vi "narrowband_response.vi"() -> ()   [LabVIEW 2012]
uses:
  Trace controls.ctl
  probe_point.ctl
  <vilib>/Analysis/4window.llb/windowTd.ctl
  stimulus.ctl
  injection_point.ctl
  pose_selector.ctl
  pose_source.ctl
  pose_relative_to.ctl
  scan_info.ctl
  <vilib>/Platform/TimedLoop/XDataNode/timing_clust.ctl
  <vilib>/Platform/TimedLoop/XDataNode/nitl_modes.ctl
  <vilib>/Platform/TimedLoop/XDataNode/wakeup.ctl
  initialization/micron_globals.vi
  <vilib>/Analysis/0measdsp.llb/Scaled Time Domain Window (DBL).vi
  <vilib>/Analysis/2dsp.llb/Real FFT.vi
  <vilib>/Analysis/2dsp.llb/Inverse Real FFT.vi
  <vilib>/Platform/TimedLoop/XDataNode/XDataNode.xnode
  <vilib>/Platform/TimedLoop/XDataNode/XDNodeRunTimeDep.lvlib
  <vilib>/Analysis/NI_AALPro.lvlib
  <vilib>/Analysis/4window.llb/Window Properties by Name.vi
  <vilib>/Analysis/4window.llb/Blackman-Harris Window (DBL).vi
panel:
  in  "Pose selectors":T1[](array[typedef])
  in  "Unwrap phase":bool=TRUE
  in  "Responses":cluster{"Individual":bool, "Vector sum":bool}={"Individual"=FALSE, "Vector sum"=TRUE}
  out "Stimulus":T4={"Type"=enum."Off", "Phase"=0.0, "Amplitude"=[0.0, 0.0, 0.0, 0.0, 0.0, 0.0], "Injection point"=enum."Total pose", "Closed loop"=FALSE, "Offset"=[0.0, 0.0, 0.0, 0.0, 0.0, 0.0], "Tip -> world"=TRUE, "Frequency"=0.0, "Length"=0.0} {"Length" min=0.0 max=100.0 step=100.0 format="%#_4p"; "Frequency" min=0.0 step=100.0 format="%#_4g"; "Offset" format="%#_3p"; "Amplitude" format="%#_3p"; "Phase" min=-180.0 max=360.0 step=100.0 format="%#.2f"}
  in  "Clear plot":bool
  out "Phase plot":T6(graph)
  out "Amplitude plot":cluster{"X out":dbl[], dbl[]}[](graph)
  out "dB re. 1 um peak":dbl caption="dB re. 1mm peak" format="%#_3f"
  out "Amplitude dB":dbl caption="dB" format="%#_3f"
  out "RMS":dbl format="%#_3p"
  out "Phase":dbl format="%#.2f"
  out "THD":dbl format="%#_4p"
  in  "N harmonics":i32=10 min=1 max=100
  out "Amplitudes":cluster{dbl, i32, dbl}[](array[cluster]) {"?" format="%#.1f"; "?" format="%#_4g"}
  in  "stop":bool
  out "Vector sum":sgl format="%#_3p"
  out "RMS":sgl[](array[numeric]) format="%#_3p"
  out "Spectrum":waveform(sgl)[](graph)
  in  "Reference":bool
  in  "Window":T7 items=["Rectangle"=0, "Hanning"=1, "Hamming"=2, "Blackman-Harris"=3, "Exact Blackman"=4, "Blackman"=5, "Flat Top"=6, "4 Term B-Harris "=7, "7 Term B-Harris"=8, "Low Sidelobe"=9, "Blackman Nuttall"=11, "Triangle"=30, "Bartlett-Hanning"=31, "Bohman"=32, "Parzen"=33, "Welch"=34, "Kaiser"=60, "Dolph-Chebyshev"=61, "Gaussian"=62]
  in  "High cutoff":sgl=100.0
  out "Time domain result":waveform(sgl)[](graph)
  in  "Components":T8={"Fundamental"=TRUE, "Harmonics"=TRUE, "Noise"=FALSE}
  out "Status":string
  in  "Trace controls":T9[](array[typedef])=[{"+ stim"=FALSE, "Relative"=FALSE, "Scale"=enum."1X", "Probe point"=enum."Position (tip)", "XYZ selector"={"Boolean"=FALSE, "Boolean 2"=FALSE, "Boolean 3"=FALSE}, "To tip"=FALSE}, {"+ stim"=FALSE, "Relative"=FALSE, "Scale"=enum."1X", "Probe point"=enum."Position (tip)", "XYZ selector"={"Boolean"=FALSE, "Boolean 2"=FALSE, "Boolean 3"=FALSE}, "To tip"=FALSE}, {"+ stim"=FALSE, "Relative"=FALSE, "Scale"=enum."1X", "Probe point"=enum."Position (tip)", "XYZ selector"={"Boolean"=FALSE, "Boolean 2"=FALSE, "Boolean 3"=FALSE}, "To tip"=FALSE}, {"+ stim"=FALSE, "Relative"=FALSE, "Scale"=enum."1X", "Probe point"=enum."Position (tip)", "XYZ selector"={"Boolean"=FALSE, "Boolean 2"=FALSE, "Boolean 3"=FALSE}, "To tip"=FALSE}]
  # "Fundamental"
  # "dB"
  # "Harmonic"
  # "Hz"
  # "Harmonics"
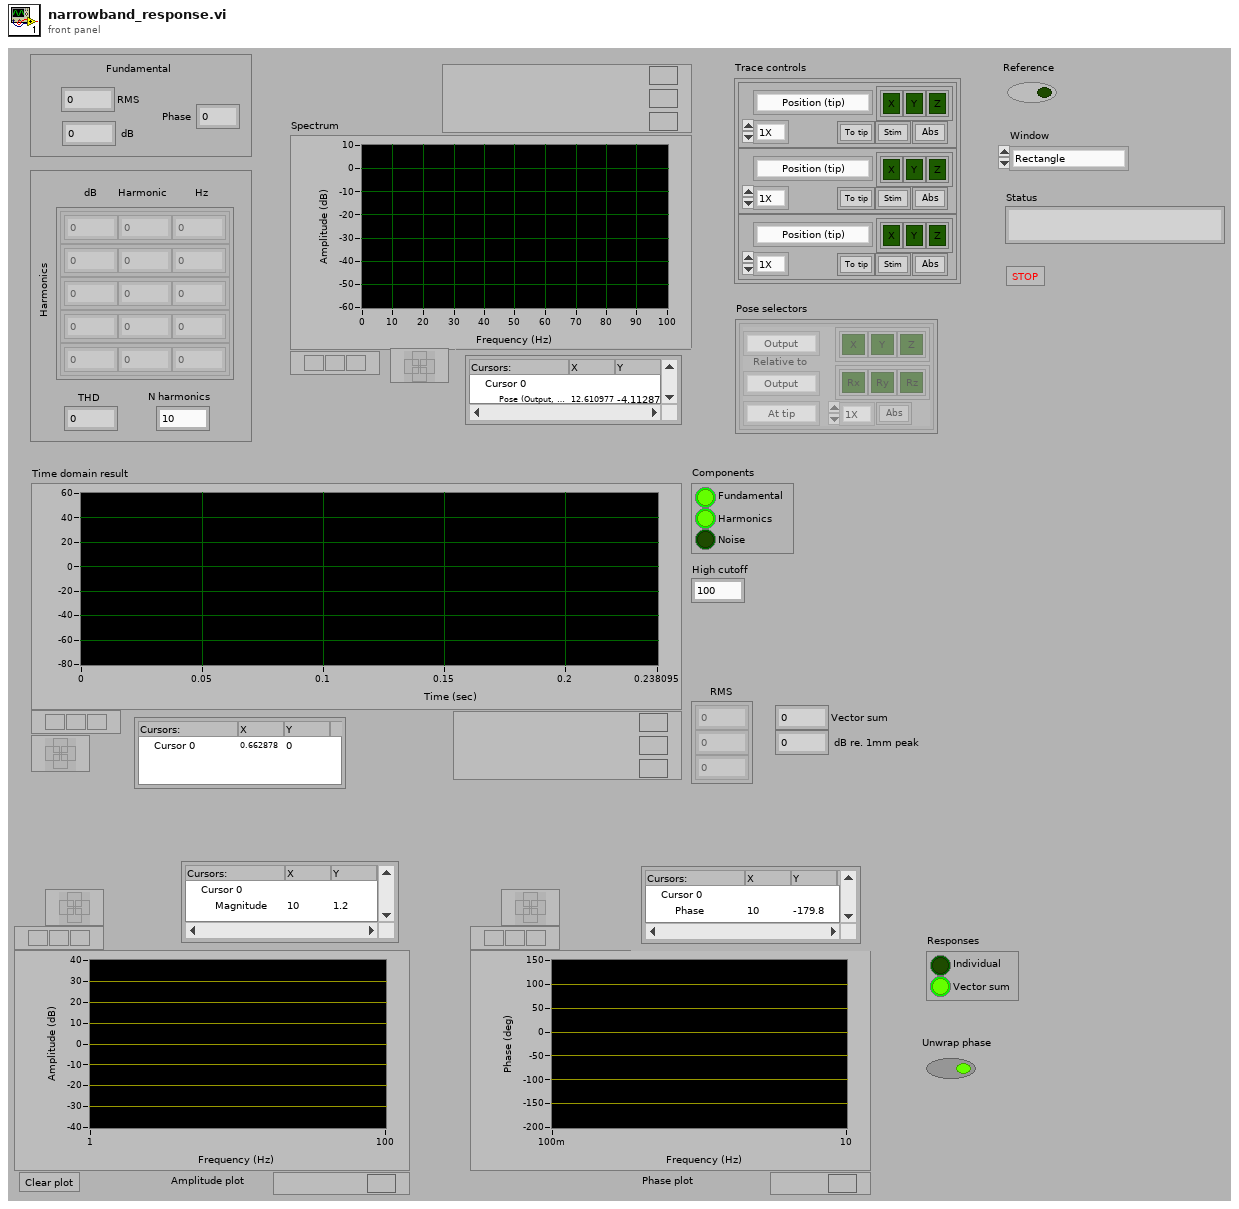
[diagram p1: front panel]
types:
  T1 = typedef "pose_selector.ctl" = cluster{"Scale":enum16{"1X", "10X", "100X", "1KX", "10KX"}, "Source":T2, "XYZ selector":cluster{"Boolean":bool, "Boolean 2":bool, "Boolean 3":bool}, "RPY selector":cluster{"Boolean":bool, "Boolean 2":bool, "Boolean 3":bool}, "Relative to":T3, "Relative":bool, "Translate":enum16{"At tip", "At RCM", "At KC", "At origin"}}
  T2 = typedef "pose_source.ctl" = enum16{"Output", "Handle", "Handle KF", "Goal", "Absolute"}
  T3 = typedef "pose_relative_to.ctl" = enum16{"Output", "Handle", "Handle KF", "Goal", "Absolute", "Trace start"}
  T4 = typedef "stimulus.ctl" = cluster{"Type":enum16{"Off", "Step", "Sine", "Triangle", "Arbitrary"}, "Phase":dbl, "Amplitude":sgl[], "Injection point":T5, "Closed loop":bool, "Offset":sgl[], "Tip -> world":bool, "Frequency":dbl, "Length":dbl}
  T5 = typedef "injection_point.ctl" = enum16{"Total pose", "V limiter", "Goal ", "Link position", "KF link position", "Inverse kin", "Link goal", "Link error", "Controller", "Output", "Drive", "Light"}
  T6 = cluster{"X out":dbl[], "Unwrapped Phase":dbl[]}[]
  T7 = typedef "NI_AALPro.lvlib/windowTd.ctl" = u32
  T8 = cluster{"Fundamental":bool, "Harmonics":bool, "Noise":bool}
  T9 = typedef "Trace controls.ctl" = cluster{"+ stim":bool, "Relative":bool, "Scale":enum16{"1X", "10X", "100X", "1KX", "10KX"}, "Probe point":T10, "XYZ selector":cluster{"Boolean":bool, "Boolean 2":bool, "Boolean 3":bool}, "To tip":bool}
  T10 = typedef "probe_point.ctl" = enum16{"Position (tip)", "Position (RCM)", "Null pos (tip)", "Null pos (RCM)", "V limiter (tip)", "V Limiter (RCM)", "Goal (tip)", "Goal (RCM)", "Link pos 0", "Link pos 1", "KF link pos 0", "KF link pos 1", "Link rate 0", "Link rate 1", "Link residue 0", "Link residue 1", "Link goal 0", "Link goal 1", "Rate limit 0", "Rate limit 1", "Link error 0", "Link error 1", "Controller 0", "Controller 1", "Output 0", "Output 1", "Drive 0", "Drive 1", "Stimulus 0", "Stimulus 1", "Trace data 0", "Trace data 1", "Analog data 0", "Analog data 1", "Status flags", "Light 0", "Light 1", "Light 2", "Light 3", "Light 4", "Light 5", "Goal origin", "Goal rotation 0", "Goal rotation 1", "Goal rotation 2", "Output origin", "Output rotation 0", "Output rotation 1", "Output rotation 2", "Handle origin", "Handle rotation 0", "Handle rotation 1", "Handle rotation 2", "Handle position", "Handle velocity", "Handle acceleration", "Handle angles", "Handle angle rates", "Handle pos residue", "Handle angle residue", "Trace length"}
  T11 = typedef "scan_info.ctl" = cluster{"Type":enum16{"Frequency", "Offset", "Motion"}, "Start":sgl, "End":sgl, "Npoints":i32}
  T12 = typedef "Micron params.ctl" = cluster{"Stimulus":T4, "Goal Filter A":T13, "Mode controls":T14, "Manipulator type":enum16{"Current piezo", "Voltage piezo"}, "Manipulator calibration":T15, "Network":T17, "Goal Filter B":T13, "Cancellation":T18, "Transition time":sgl, "Estimation":T20}
  T13 = typedef "goal_loop_parms.ctl" = cluster{"Speedup max":sgl, "Speedup thresh":sgl, "Speedup nonlin":sgl, "Filters":cluster{"Lower Fc":sgl, "Lower Q":sgl, "Scale factor":sgl, "Upper Fc":sgl, "Upper Q":sgl, "V limit":sgl, "V limit range":sgl}[]}
  T14 = typedef "mode_conrols.ctl" = cluster{"Hold":bool, "Cancellation":bool, "Goal filter":bool, "Trigger":bool}
  T15 = typedef "manipulator_cal.ctl" = cluster{"Tool offsets":sgl[][], "Tip light calibration":T16, "Handle light calibration":T16, "Base pivots":sgl[][], "Output pivots":sgl[][], "Length center":sgl, "Workspace height":sgl[], "Workspace diameter":sgl[], "Linearization":sgl[][], "Stack travel":sgl, "Saturation pos":sgl, "Inverse filters":cluster{"filter structure":enum32{"IIR 2nd Order", "IIR 4th Order"}, "Reverse Coefficients":dbl[], "Forward Coefficients":dbl[]}[]}
  T16 = typedef "probe_calibration.ctl" = sgl[][]
  T17 = typedef "network_params.ctl" = cluster{"Remote Host":string, "Send Status":bool, "Send Port":u16, "Recv Commands":bool, "Recv Port":u16}
  T18 = typedef "sq_control_params.ctl" = cluster{"KP":T19, "KI":sgl, "KD":T19, "Max vel":sgl, "Max acc":sgl, "Int error limit":sgl, "RCM gain":sgl, "Bypass":bool, "Degraded gain":sgl}
  T19 = typedef "decoupled_gain.ctl" = cluster{"XY":sgl, "Rxy":sgl, "Z":sgl, "Rz":sgl}
  T20 = typedef "estimation_controls.ctl" = cluster{"Link":cluster{"Measure noise":dbl[], "Process noise":dbl[], "Alt process noise":dbl[], "Alt turnoff cycles":i32, "Innovation limit":dbl[], "Residue threshold":dbl, "Enable":bool}, "Handle":cluster{"Measure noise":dbl[], "Process noise":dbl[], "State limits":dbl[], "Innovation limit":dbl[], "Prediction Lookahead":sgl, "Enable":bool}}
  T21 = typedef "XDNodeRunTimeDep.lvlib/timing_clust.ctl" = cluster{"Expected End [f-1]":u64, "Actual End [f-1]":u64, "Finished Late? [f-1]":bool, "Expected End [i-1]":u64, "Actual End [i-1]":u64, "Finished Late? [i-1]":bool, "Expected Start [i]":u64, "Actual Start [i]":u64, "Expected Start [f]":u64, "Actual Start [f]":u64, "Source Name":string, "Structure Name":string, "Period":i64, "Deadline":i64, "Offset":i64, "Start":i64, "Priority":i32, "Timeout":i32, "Mode":T22, "Wakeup Reason":T23, "Error":errorcluster, "Source Type":string, "Secondary Source Type":string, "Global End Time":u64, "Global Start Time":u64, "Frame Duration":u64, "Iteration Duration":u64, "Assigned CPU":i32, "I/O Scan Engine Mode":u32}
  T22 = typedef "XDNodeRunTimeDep.lvlib/nitl_modes.ctl" = enum32{"No Change", "Process missed periods, maintain original phase", "Discard missed periods, maintain original phase", "Process missed periods, ignore original phase", "Discard missed periods, ignore original phase"}
  T23 = typedef "XDNodeRunTimeDep.lvlib/wakeup.ctl" = enum32{"Normal", "Aborted", "Asynchronous wakeup", "Timing source error", "Timed loop error", "Timeout"}
  T24 = cluster{"Components":cluster{"Fundamental":bool, "Harmonics":bool, "Noise":bool}, "High cutoff":sgl, "N harmonics":i32, "Reference":bool, "Window":T7}
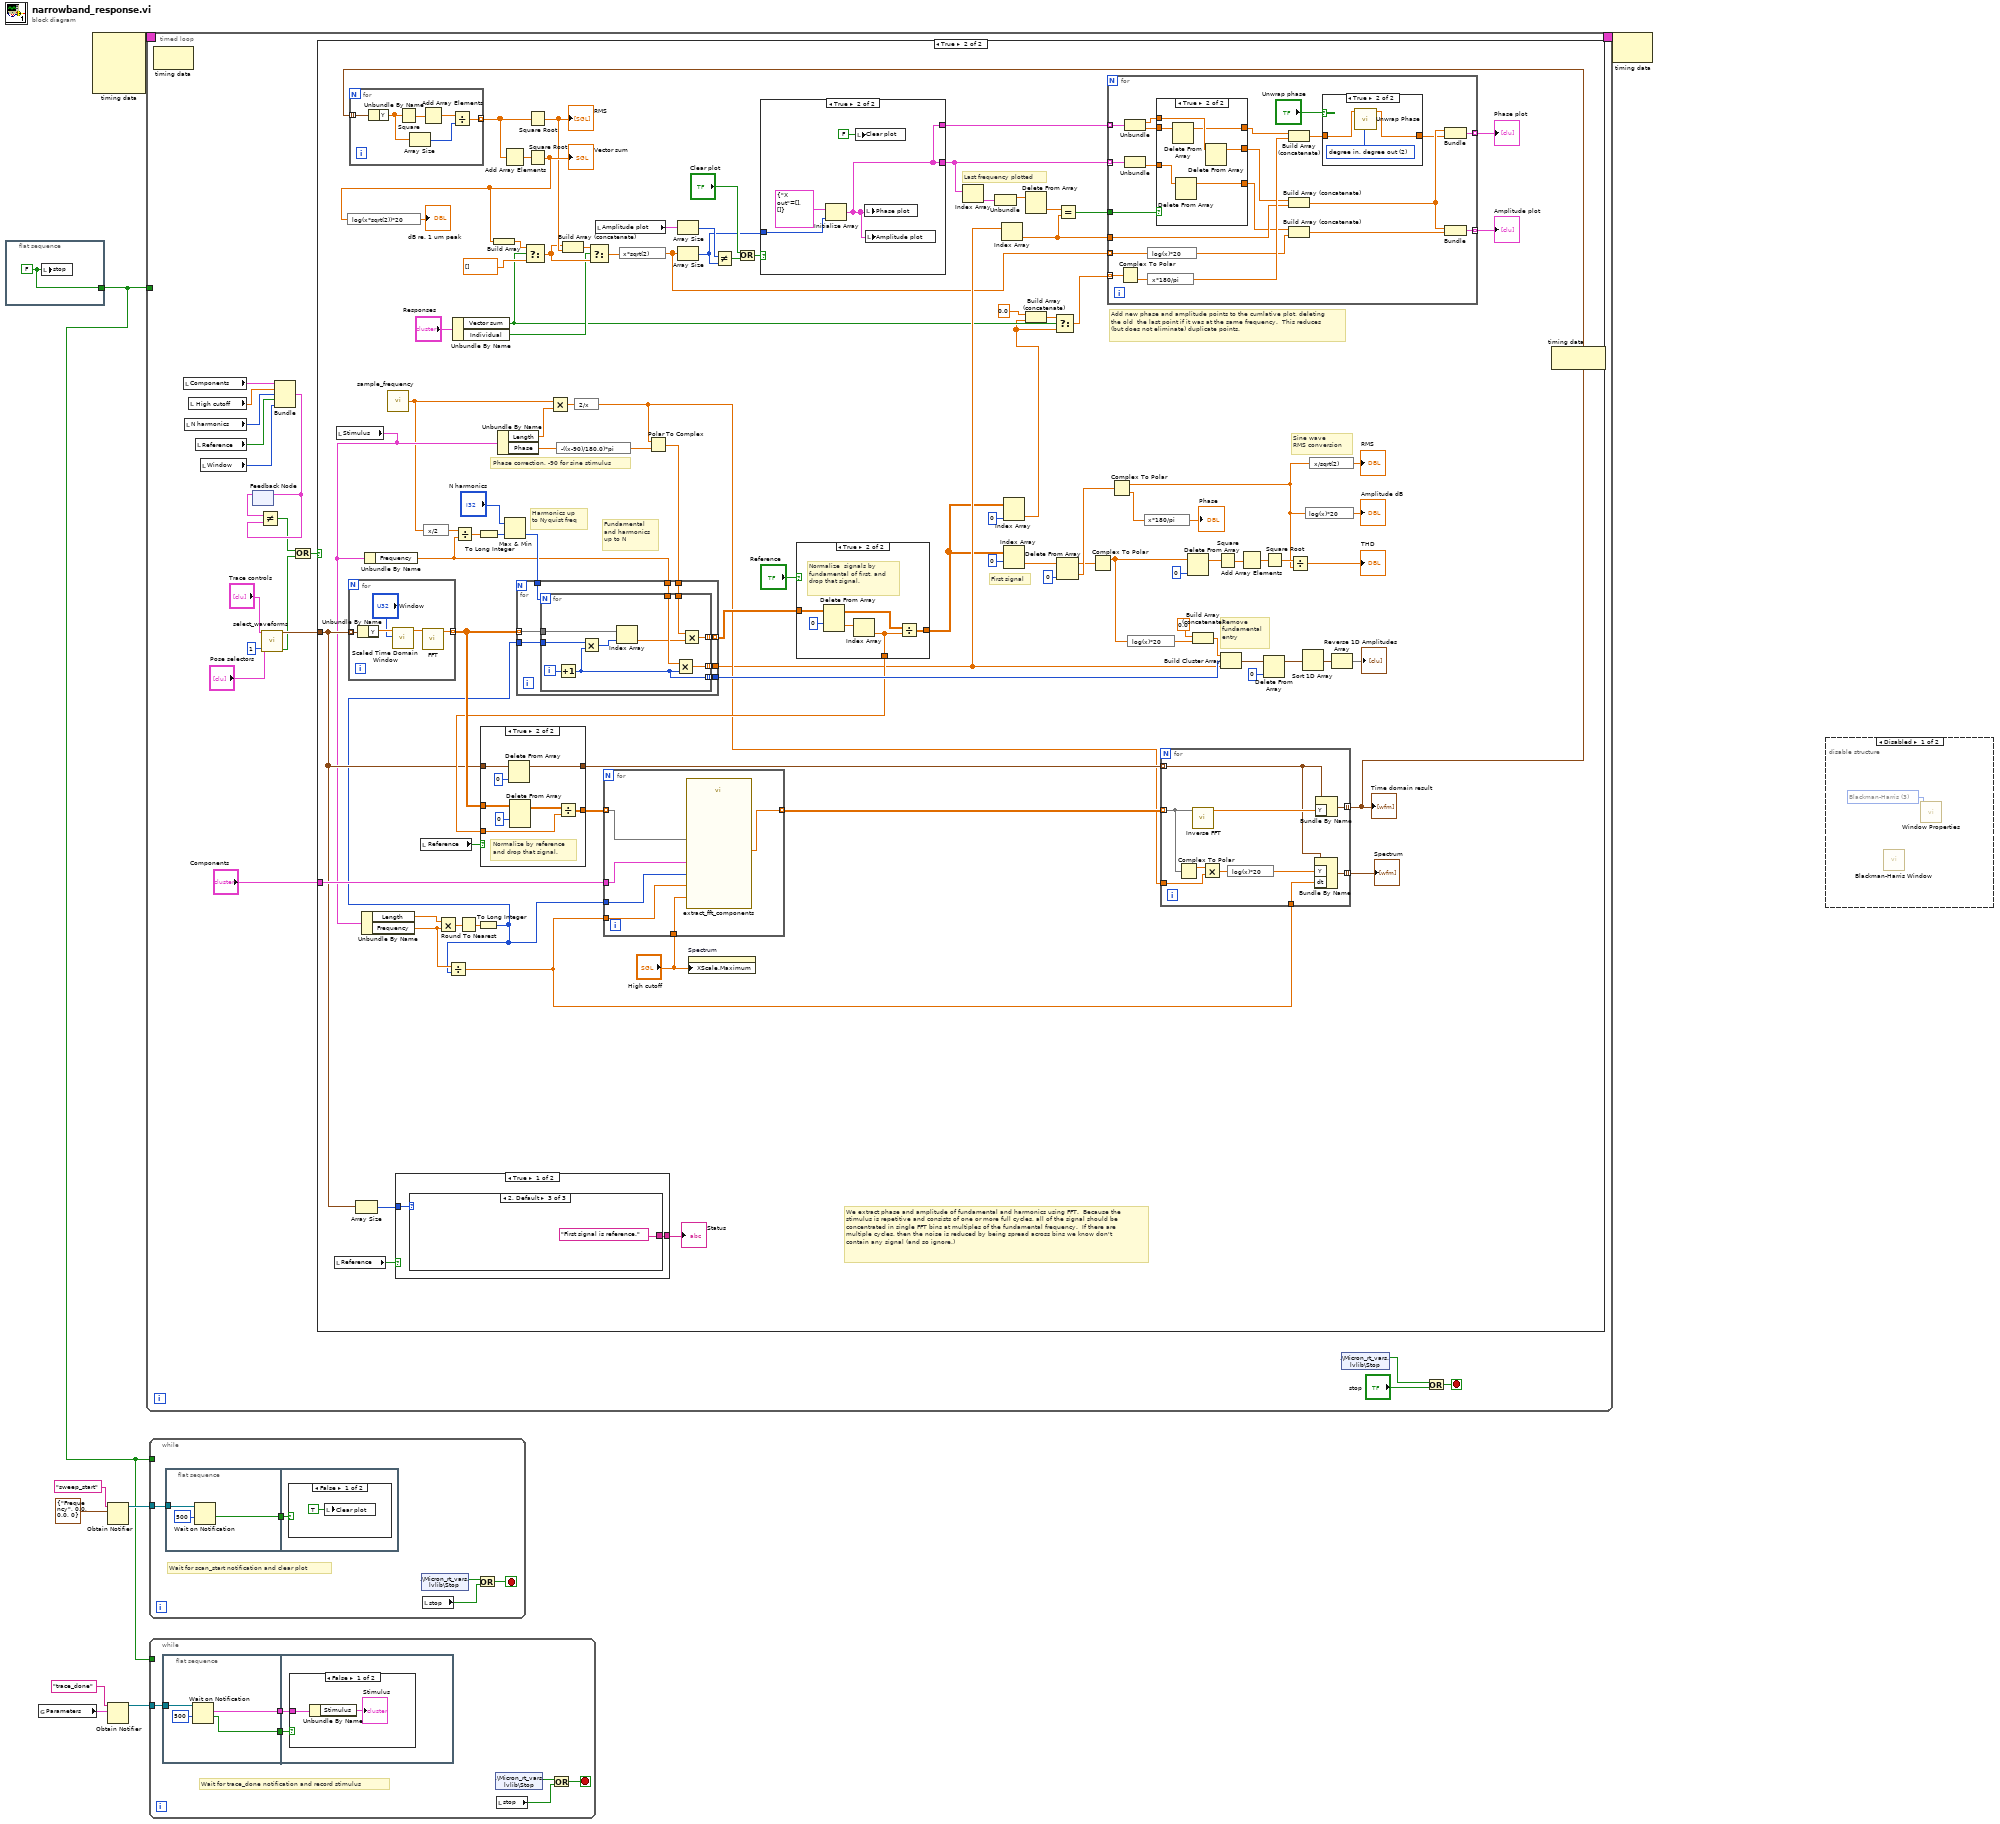
[diagram p0: block diagram]
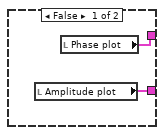
[diagram p8: hidden frame]
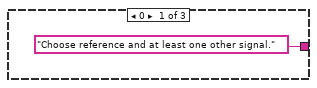
[diagram p10: hidden frame]
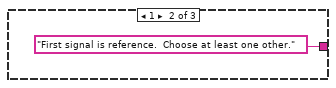
[diagram p11: hidden frame]
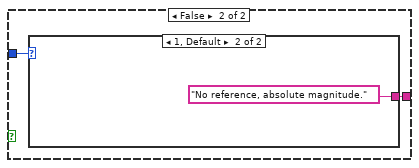
[diagram p12: hidden frame]
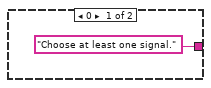
[diagram p13: hidden frame]
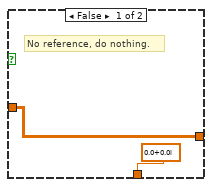
[diagram p14: hidden frame]
diagram:
  n1 = flat-sequence {
    tunnel: [w10] -> w1
    frame #0 {
      w10 = FALSE ("stop")
      n2 = local write "stop"(w10) -> ()
    }
  }
  n3 = global read "micron_globals.vi" "Parameters"() -> (w2:T12)
  n4 = node-c288() -> (w9:T21)  [unwired: 4 out]
  n5 = Obtain Notifier(name (unnamed)="sweep_start", notification data type=T11 {"Type"=enum."Frequency", "Start"=0.0, "End"=0.0, "Npoints"=0} ("Scan Info")) -> (notifier out=w5:refnum<notifier>)  [unwired: 2 in, 2 out]
  n6 = Obtain Notifier(name (unnamed)="trace_done", notification data type=w2) -> (notifier out=w4:refnum<notifier>)  [unwired: 2 in, 2 out]
  n7 = timed-loop {
    timing: w9 -> [_]
    timing-out: [_] -> w8
    tunnel: w1 -> [_]
    stop <- w22 stop-if-true
    n8 = node-c288() -> ()  [unwired: 2 out]
    n9 = local read "Components"() -> (w16:T8)
    n10 = local read "N harmonics"() -> (w14:i32)
    n11 = local read "High cutoff"() -> (w15:sgl)
    n12 = local read "Reference"() -> (w13:bool)
    n13 = local read "Window"() -> (w12:T7)
    n14 = feedback #1() -> (w25:T24)  [unwired: 1 in]
    n15 = call "select_waveforms.vi"("Trace controls"="Trace controls", "Pose selectors"="Pose selectors", "Decimate"=1) -> ("Waveforms out"=w26:waveform(sgl)[], "New data"=w18:bool)  [unwired: 9 in, 2 out]
    n16 = Bundle("Components"=w16, "High cutoff"=w15, "N harmonics"=w14, "Reference"=w13, "Window"=w12) -> (w19:T24)  [unwired: 1 in]
    n17 = feedback-in #1(w19) -> ()
    n18 = Not Equal?(x=w25, y=w19) -> (x != y?=w17:bool)
    n19 = Or(x=w17, y=w18) -> (x .or. y?=w23:bool)
    n20 = case shown="True" w23 {
      tunnel: w26 -> [_ w77]
      tunnel: "Components" -> [_ w92]
      frame False {
      }
      frame True {
        # "First signal"
        # "We extract phase and amplitude of fundamental and harmonics using FFT.  Because the stimulus is repetitive and consists of one or more full cycles, all of the signal should be concentrated in single FFT bins at multiples of the fundamental frequency.  If there are multiple cycles, then the noise is reduced by being spread across bins we know don't contain any signal (and so ignore.)"
        # "Add new phase and amplitude points to the cumlative plot, deleting the old  the last point if it was at the same frequency.  This reduces (but does not eliminate) duplicate points."
        # "Last frequency plotted"
        # "Sine wave\nRMS conversion"
        # "Fundamental and harmonics up to N"
        # "Remove\nfundamental\nentry"
        # "Harmonics up\nto Nyquist freq"
        # "Phase correction, -90 for sine stimulus"
        n21 = local read "Reference"() -> (w87:bool)
        n22 = local read "Stimulus"() -> (w51:T4)
        n23 = for {
          tunnel: w77 -> [w213] mode=indexing
          tunnel: [w212] -> w126 mode=indexing
          n24 = Unbundle By Name(w213) -> ("Y"=w211:sgl[])
          n25 = call-poly <vilib>:"Scaled Time Domain Window.vi"("window"="Window", "X"=w211) -> ("Windowed X"=w210:dbl[])  [unwired: 7 in, 2 out]
          n26 = call-poly <vilib>:"FFT.vi"("X"=w210) -> ("FFT {X}"=w212:cdb[])  [unwired: 9 in, 1 out]
        }
        n27 = Array Size(array=w77) -> (size(s)=w86:i32)
        n28 = Unbundle By Name(w51) -> ("Length"=w90:dbl, "Frequency"=w89:dbl)
        n29 = Unbundle By Name(w51) -> ("Frequency"=w91:dbl)
        n30 = call "sample_frequency.vi"() -> ("Sample frequency"=w32:dbl)
        n31 = case shown="True" w87 {
          tunnel: [w185 w190] -> w93
          tunnel: w86 -> [w184 w189]
          frame True {
            n32 = case shown="2, Default" w184 {
              tunnel: ["Choose reference and at least one other signal." ("message") "First signal is reference.  Choose at least one other." ("message") "First signal is reference." ("message")] -> w185
              frame 0 {
              }
              frame 1 {
              }
              frame 2, Default {
              }
            }
          }
          frame False {
            n33 = case shown="1, Default" w189 {
              tunnel: ["Choose at least one signal." ("message") "No reference, absolute magnitude." ("message")] -> w190
              frame 0 {
              }
              frame 1, Default {
              }
            }
          }
        }
        "Status" <- w93
        n34 = local read "Reference"() -> (w84:bool)
        n35 = expression code="x/2"(w32) -> (w125:dbl)
        n36 = Multiply(x=w90, y=w89) -> (x*y=w122:dbl)
        n37 = Unbundle By Name("Responses") -> ("Vector sum"=w38:bool, "Individual"=w42:bool)
        n38 = Divide(x=w125, y=w91) -> (x/y=w124:dbl)
        n39 = Round To Nearest(number=w122) -> (nearest integer value=w121:dbl)
        n40 = To Long Integer(number=w121) -> (32bit integer=w30:i32)
        n41 = Divide(x=w89, y=w30) -> (x/y=w79:dbl)
        n42 = To Long Integer(number=w124) -> (32bit integer=w112:i32)
        n43 = Unbundle By Name(w51) -> ("Length"=w33:dbl, "Phase"=w119:dbl)
        n44 = Max & Min(x="N harmonics", y=w112) -> (min(x,y)=w111:i32)  [unwired: 1 out]
        n45 = Multiply(x=w32, y=w33) -> (x*y=w31:dbl)
        n46 = expression code="-((x-90)/180.0)*pi" ("degrees to radians")(w119) -> (w123:dbl)
        n47 = expression code="2/x" ("degrees to radians")(w31) -> (w76:dbl)
        n48 = local read "Amplitude plot"() -> (w67:cluster{"X out":dbl[], dbl[]}[])
        n49 = Polar To Complex(1:w123, 2:w76) -> (0:w120:cdb)
        n50 = for {
          tunnel: w111 -> [w221]
          tunnel: w91 -> [w220]
          tunnel: w30 -> [w215]
          tunnel: w120 -> [w219]
          tunnel: [w218] -> w118 mode=indexing
          tunnel: [w217] -> w61
          tunnel: [w216] -> w116
          tunnel: w126 -> [w214] mode=indexing
          n51 = for {
            N: w221 -> [_]
            tunnel: w214 -> [w231]
            tunnel: w220 -> [w230]
            tunnel: w215 -> [w229]
            tunnel: w219 -> [w228]
            tunnel: [w226] -> w218 mode=indexing
            tunnel: [w227] -> w217 mode=indexing
            tunnel: [w224] -> w216 mode=indexing
            i -> [w225]
            n52 = Increment(x=w225) -> (x+1=w224:i32)
            n53 = Multiply(x=w229, y=w224) -> (x*y=w223:i32)
            n54 = Index Array(array=w231, index=w223) -> (element=w222:cdb)
            n55 = Multiply(x=w230, y=w224) -> (x*y=w227:dbl)
            n56 = Multiply(x=w228, y=w222) -> (x*y=w226:cdb)
          }
        }
        n57 = Array Size(array=w67) -> (size(s)=w66:i32)
        n58 = property on="Spectrum" class="WFGraph (strict)"("XScale.Maximum"="High cutoff") -> ()  [unwired: 2 in, 2 out]
        n59 = case shown="True" "Reference" {
          tunnel: w118 -> [w232 w238]
          tunnel: [w232 w235] -> w60
          tunnel: [cdb 0.0+0.0i w234] -> w82
          frame False {
            # "No reference, do nothing."
          }
          frame True {
            # "Normalize  signals by fundamental of first, and drop that signal."
            n60 = Delete From Array(array=w238, index (row)=0 ("length")) -> (deleted portion=w237:cdb[], array with subset deleted=w236:cdb[][])  [unwired: 2 in]
            n61 = Index Array(array=w237) -> (element=w234:cdb)  [unwired: 1 in]
            n62 = Divide(x=w236, y=w234) -> (x/y=w235:cdb[][])
          }
        }
        n63 = case shown="True" w84 {
          tunnel: w126 -> [w175 w183]
          tunnel: [w175 w181] -> w83
          tunnel: w82 -> [_ w179]
          tunnel: [w174 w176] -> w78
          tunnel: w77 -> [w174 w178]
          frame False {
            # "No reference, just pass\nthrough."
          }
          frame True {
            # "Normalize by reference\nand drop that signal."
            n64 = Delete From Array(array=w178, index=0) -> (array with subset deleted=w176:waveform(sgl)[])  [unwired: 1 in, 1 out]
            n65 = Delete From Array(array=w183, index (row)=0 ("length")) -> (array with subset deleted=w180:cdb[][])  [unwired: 2 in, 1 out]
            n66 = Divide(x=w180, y=w179) -> (x/y=w181:cdb[][])
          }
        }
        n67 = for {
          tunnel: w30 -> [w208]
          tunnel: w83 -> [w207] mode=indexing
          tunnel: w92 -> [w206]
          tunnel: [w205] -> w81 mode=indexing
          tunnel: w79 -> [w204]
          tunnel: "High cutoff" -> [w203]
          n68 = call "extract_fft_components.vi"("Freq resolution"=w204, "High cutoff"=w203, "Cycles in block"=w208, "Components"=w206, "FFT {X} in"=w207) -> ("FFT {X} out"=w205:cdb[])  [unwired: 6 in]
        }
        n69 = Index Array(array=w61) -> (element=w54:dbl)  [unwired: 1 in]
        n70 = Index Array(array=w60, index (col)=0 ("disabled index (col)")) -> (element=w37:cdb[])  [unwired: 1 in]
        n71 = Index Array(array=w60, index (row)=0) -> (element=w68:cdb[])  [unwired: 1 in]
        n72 = Build Array (concatenate)(0.0, w37) -> (w35:cdb[])
        n73 = Select(t=w35, s=w38, f=w37) -> (s? t:f=w36:cdb[])
        n74 = Delete From Array(array=w68, index=0) -> (deleted portion=w100:cdb, array with subset deleted=w85:cdb[])  [unwired: 1 in]
        n75 = Complex To Polar(r * e^(i*theta)=w85) -> (r=w101:dbl[])  [unwired: 1 out]
        n76 = Complex To Polar(r * e^(i*theta)=w100) -> (r=w72:dbl, theta=w104:dbl)
        n77 = expression code="log(x)*20"(w101) -> (w99:dbl[])
        n78 = expression code="x*180/pi"(w104) -> (→"Phase":dbl)
        n79 = for {
          tunnel: w78 -> [w200] mode=indexing
          tunnel: w81 -> [w197] mode=indexing
          tunnel: [w201] -> w75 mode=indexing
          tunnel: [w199] -> w80 mode=indexing
          tunnel: w79 -> [w198]
          tunnel: w76 -> [w195]
          n80 = Complex To Polar(r * e^(i*theta)=w197) -> (r=w196:dbl[])  [unwired: 1 out]
          n81 = call-poly <vilib>:"Inverse FFT.vi"("FFT {X}"=w197) -> ("X"=w202:dbl[])  [unwired: 9 in, 1 out]
          n82 = Multiply(x=w196, y=w195) -> (x*y=w194:dbl[])
          n83 = expression code="log(x)*20"(w194) -> (w193:dbl[])
          n84 = Bundle By Name(cluster=w200, "Y"=w193, "dt"=w198) -> (w199:waveform(sgl))
          n85 = Bundle By Name(cluster=w200, "Y"=w202) -> (w201:waveform(sgl))
        }
        "Time domain result" <- w75
        "Spectrum" <- w80
        n86 = for {
          tunnel: w75 -> [w173] mode=indexing
          tunnel: [w168] -> w74 mode=indexing
          n87 = Unbundle By Name(w173) -> ("Y"=w170:sgl[])
          n88 = Square(x=w170) -> (x^2=w172:sgl[])
          n89 = Array Size(array=w170) -> (size(s)=w169:i32)
          n90 = Add Array Elements(numeric array=w172) -> (sum=w171:sgl)
          n91 = Divide(x=w171, y=w169) -> (x/y=w168:sgl)
        }
        n92 = Add Array Elements(numeric array=w74) -> (sum=w71:sgl)
        n93 = Square Root(x=w74) -> (sqrt(x)=w44:sgl[])
        "RMS" <- w44
        n94 = Square Root(x=w71) -> (sqrt(x)=w46:sgl)
        "Vector sum" <- w46
        n95 = expression code="log(x*sqrt(2))*20"(w46) -> (→"dB re. 1 um peak":sgl)
        n96 = Build Array(w46) -> (w47:sgl[])
        n97 = Select(t=w47, s=w38, f=sgl[] [] ("appended array")) -> (s? t:f=w43:sgl[])
        n98 = Build Array (concatenate)(w43, w44) -> (w45:sgl[])
        n99 = Select(t=w45, s=w42, f=w43) -> (s? t:f=w41:sgl[])
        n100 = expression code="x*sqrt(2)"(w41) -> (w39:sgl[])
        n101 = Array Size(array=w39) -> (size(s)=w40:i32)
        n102 = Not Equal?(x=w66, y=w40) -> (x != y?=w65:bool)
        n103 = Or(x="Clear plot", y=w65) -> (x .or. y?=w64:bool)
        n104 = case shown="True" w64 {
          tunnel: w40 -> [_ w166]
          tunnel: [w163 w164] -> w57
          tunnel: [w162 w164] -> w56
          frame False {
            n105 = local read "Amplitude plot"() -> (w163:cluster{"X out":dbl[], dbl[]}[])
            n106 = local read "Phase plot"() -> (w162:T6)
          }
          frame True {
            n107 = Initialize Array(cluster{"X out":dbl[], dbl[]} {"X out"=[], []}, w166) -> (w164:cluster{"X out":dbl[], dbl[]}[])
            n108 = local write "Clear plot"(FALSE ("Clear plot")) -> ()
            n109 = local write "Phase plot"(w164) -> ()
            n110 = local write "Amplitude plot"(w164) -> ()
          }
        }
        n111 = Index Array(array=w57) -> (element=w63:cluster{"X out":dbl[], dbl[]})  [unwired: 1 in]
        n112 = Unbundle(w63) -> ("X out"=w62:dbl[])  [unwired: 1 out]
        n113 = Delete From Array(array=w62) -> (deleted portion=w58:dbl)  [unwired: 2 in, 1 out]
        n114 = Equal?(x=w58, y=w54) -> (x = y?=w55:bool)
        n115 = for {
          tunnel: w36 -> [w147] mode=indexing
          tunnel: w57 -> [w146] mode=indexing
          tunnel: w56 -> [w145] mode=indexing
          tunnel: w55 -> [w142]
          tunnel: w54 -> [w141]
          tunnel: [w136] -> w53 mode=indexing
          tunnel: [w133] -> w52 mode=indexing
          tunnel: w39 -> [w130] mode=indexing
          n116 = Complex To Polar(r * e^(i*theta)=w147) -> (theta=w148:dbl)  [unwired: 1 out]
          n117 = Unbundle(w145) -> ("X out"=w131:dbl[], "Unwrapped Phase"=w132:dbl[])
          n118 = Unbundle(w146) -> (w138:dbl[])  [unwired: 1 out]
          n119 = expression code="log(x)*20"(w130) -> (w143:sgl)
          n120 = expression code="x*180/pi"(w148) -> (w144:dbl)
          n121 = case shown="True" w142 {
            tunnel: w132 -> [w155 w161]
            tunnel: w131 -> [w154 w160]
            tunnel: [w155 w159] -> w140
            tunnel: [w154 w158] -> w139
            tunnel: w138 -> [w153 w157]
            tunnel: [w153 w156] -> w137
            frame False {
            }
            frame True {
              n122 = Delete From Array(array=w161) -> (array with subset deleted=w159:dbl[])  [unwired: 2 in, 1 out]
              n123 = Delete From Array(array=w157) -> (array with subset deleted=w156:dbl[])  [unwired: 2 in, 1 out]
              n124 = Delete From Array(array=w160) -> (array with subset deleted=w158:dbl[])  [unwired: 2 in, 1 out]
            }
          }
          n125 = Build Array (concatenate)(w140, w144) -> (w128:dbl[])
          n126 = Build Array (concatenate)(w139, w141) -> (w134:dbl[])
          n127 = Build Array (concatenate)(w137, w143) -> (w135:dbl[])
          n128 = case shown="True" "Unwrap phase" {
            tunnel: [w149 w150] -> w129
            tunnel: w128 -> [w149 w151]
            frame False {
            }
            frame True {
              w152 = 2 items=["radian in, radian out", "radian in, degree out", "degree in, degree out", "degree in, radian out"] ("phase unit")
              n129 = call <vilib>:"Unwrap Phase.vi"("phase unit"=w152, "Phase"=w151) -> ("Unwrapped Phase"=w150:dbl[])  [unwired: 8 in, 1 out]
            }
          }
          n130 = Bundle(w134, "Unwrapped Phase"=w129) -> (w136:cluster{dbl[], "Unwrapped Phase":dbl[]})  [unwired: 1 in]
          n131 = Bundle(w134, w135) -> (w133:cluster{dbl[], dbl[]})  [unwired: 1 in]
        }
        "Amplitude plot" <- w52
        "Phase plot" <- w53
        n132 = Delete From Array(array=w101, index=0) -> (array with subset deleted=w103:dbl[])  [unwired: 1 in, 1 out]
        n133 = Build Array (concatenate)(0.0 ("x/y"), w99) -> (w98:dbl[])
        n134 = Square(x=w103) -> (x^2=w109:dbl[])
        n135 = Build Cluster Array(w98, w116, w61) -> (w95:cluster{"x/y":dbl, i32, dbl}[])
        n136 = Add Array Elements(numeric array=w109) -> (sum=w108:dbl)
        n137 = Delete From Array(array=w95, index=0) -> (array with subset deleted=w94:cluster{"x/y":dbl, i32, dbl}[])  [unwired: 1 in, 1 out]
        n138 = Square Root(x=w108) -> (sqrt(x)=w107:dbl)
        n139 = Divide(x=w107, y=w72) -> (x/y=→"THD":dbl)
        n140 = Sort 1D Array(array=w94) -> (sorted array=w115:cluster{"x/y":dbl, i32, dbl}[])
        n141 = expression code="log(x)*20"(w72) -> (→"Amplitude dB":dbl)
        n142 = expression code="x/sqrt(2)"(w72) -> (→"RMS":dbl)
        n143 = Reverse 1D Array(array=w115) -> (reversed array=→"Amplitudes":cluster{"x/y":dbl, i32, dbl}[])
      }
    }
    n144 = shared-variable ".\\Micron_rt_vars.lvlib\\Stop"() -> (w20:bool)  [unwired: 1 in, 1 out]
    n145 = Or(x=w20, y="stop") -> (x .or. y?=w22:bool)
    n146 = node-c288() -> ()  [unwired: 2 out]
  }
  n147 = while {
    tunnel: w5 -> [w246]
    tunnel: w1 -> [_]
    stop <- w243 stop-if-true
    # "Wait for scan_start notification and clear plot"
    n148 = flat-sequence {
      tunnel: w246 -> [w249]
      tunnel: [w247] -> w242
      tunnel: w242 -> [w250]
      frame #0 {
        n149 = Wait on Notification(notifier=w249, timeout in ms (-1)=500) -> (timed out?=w247:bool)  [unwired: 2 in, 3 out]
      }
      frame #1 {
        n150 = case shown="False" w250 {
          frame False {
            n151 = local write "Clear plot"(TRUE ("Clear plot")) -> ()
          }
          frame True {
          }
        }
      }
    }
    n152 = shared-variable ".\\Micron_rt_vars.lvlib\\Stop"() -> (w245:bool)  [unwired: 1 in, 1 out]
    n153 = local read "stop"() -> (w244:bool)
    n154 = Or(x=w245, y=w244) -> (x .or. y?=w243:bool)
  }
  n155 = while {
    tunnel: w4 -> [w257]
    tunnel: w1 -> [_]
    stop <- w254 stop-if-true
    # "Wait for trace_done notification and record stimulus"
    n156 = flat-sequence {
      tunnel: w257 -> [w261]
      tunnel: [w259] -> w253
      tunnel: [w258] -> w252
      tunnel: w253 -> [w263]
      tunnel: w252 -> [w262]
      frame #0 {
        n157 = Wait on Notification(notifier=w261, timeout in ms (-1)=500) -> (notification=w259:T12, timed out?=w258:bool)  [unwired: 2 in, 2 out]
      }
      frame #1 {
        n158 = case shown="False" w262 {
          tunnel: w263 -> [w265 _]
          frame False {
            n159 = Unbundle By Name(w265) -> ("Stimulus"=→"Stimulus":T4)
          }
          frame True {
          }
        }
      }
    }
    n160 = shared-variable ".\\Micron_rt_vars.lvlib\\Stop"() -> (w256:bool)  [unwired: 1 in, 1 out]
    n161 = local read "stop"() -> (w255:bool)
    n162 = Or(x=w256, y=w255) -> (x .or. y?=w254:bool)
  }
  n163 = node-c288(w8) -> ()  [unwired: 1 out]
  n164 = disable-structure shown="Disabled" {
    frame Disabled {
      w266 = T7 3 items=["Rectangle"=0, "Hanning"=1, "Hamming"=2, "Blackman-Harris"=3, "Exact Blackman"=4, "Blackman"=5, "Flat Top"=6, "4 Term B-Harris "=7, "7 Term B-Harris"=8, "Low Sidelobe"=9, "Blackman Nuttall"=11, "Triangle"=30, "Bartlett-Hanning"=31, "Bohman"=32, "Parzen"=33, "Welch"=34, "Kaiser"=60, "Dolph-Chebyshev"=61, "Gaussian"=62] ("window")
      n165 = call-poly <vilib>:"Blackman-Harris Window.vi"() -> ()  [unwired: 1 in, 2 out]
      n166 = call-poly <vilib>:"Window Properties.vi"("window"=w266) -> ()  [unwired: 8 in, 3 out]
    }
    frame Enabled {
    }
  }
